vi "Main.vi"() -> ()   [LabVIEW 2017]
doc: "This Continuous Measurement sample project is based on the Queued Message Handler template.\n\nThe Event Handling Loop generates messages based on user interface actions.\n\nThe Message Handling Loop processes messages generated by the Event Handling Loop, or by other messages. There are also Acquisition and Logging message handling loop subVIs, and a chart updating loop."
uses:
  Acquisition/Hardware Configuration.ctl
  Logging/Logging Configuration.ctl
  <vilib>/measure/madcrms.llb/Averaged DC-RMS for 1 Chan.vi
  Feedback.vi
  <vilib>/express/express analysis/Spectral/Block/exnSpectralBlock spectral measurements PSD poly.vi
  <vilib>/express/express analysis/Spectral/Block/exnSpectralBlock spectral measurements PSD DDT.vi
  support/Message Queue/Enqueue Message (Single).vi
  <vilib>/Utility/error.llb/Error Cluster From Error Code.vi
  <vilib>/express/express analysis/Spectral/XNode/ExpressSpectralMeasurementsBlockNode.xnode
  <vilib>/ErrorRing/Error Ring.xnode
  Acquisition/Acquisition.lvlib
  Logging/Logging.lvlib
  Settings/Settings.lvlib
  support/User Event - Stop/User Event - Stop.lvlib
  support/Message Queue/Message Queue.lvlib
  <vilib>/Analysis/NI_AALBase.lvlib
  <vilib>/measure/NI_MAPro.lvlib
panel:
  in  "Average_ON":bool
  in  "Clear":bool
  out "Trap_Power":dbl caption="Trap (V)"
  out "T1Y 2":waveform(dbl)(graph)={"t0"=timestamp(0 s since 1904-01-01), "dt"=1.0, "Y"=[]}
  in  "Reset":bool caption="Offset_Reset"
  out "QPD_x":dbl
  out "QPD_y":dbl
  in  "ON":bool
  in  "B1X_nm2V 2":dbl=1450.0 caption="X"
  in  "B1Y_nm2V 2":dbl=950.0 caption="Y"
  out "Fy":dbl
  out "Fx":dbl caption="F (pN)"
  in  "B1Y_stiffness":dbl=0.1 caption="B1X"
  in  "B1X_stiffness":dbl=0.1 caption="B1X"
  in  "Averaging rate (Hz)":dbl=1000.0 min=1.0 max=1000.0 step=1.0
  in  "Stiffness":bool
  out "B1X PSD":dynamicdata(graph)=[{"t0"=timestamp(0 s since 1904-01-01), "dt"=inf, "Y"=[], "attributes"=variant("NI_ChannelName"=variant(string "Collected (PSD)"), "NI_OriginalChannelName"=variant(string "Collected"))}]
  out "Logging file":path
  out "Stiffness_B1X":dbl
  out "Stiffness_B1Y":dbl
  out "B1S":waveform(dbl)(graph)={"t0"=timestamp(0 s since 1904-01-01), "dt"=1.0, "Y"=[]}
  out "B1X":waveform(dbl)(graph)
  out "B1Y":waveform(dbl)(graph)
  in  "BXY":bool
  out "B1XY":cluster{dbl[], dbl[]}(graph)
  out "T1Y":waveform(dbl)(graph)
  out "T1X":waveform(dbl)(graph)
  out "PZTZ":waveform(dbl)(graph)
  out "PZTY":waveform(dbl)(graph)
  out "PZTX":waveform(dbl)(graph)
  in  "PSD":bool
  in  "B1X_nm2V":dbl=100.0 caption="X"
  in  "B1Y_nm2V":dbl=60.0 caption="Y"
  out "Description":string
  out "User":string
  out "B1Y PSD":dynamicdata(graph)=[{"t0"=timestamp(0 s since 1904-01-01), "dt"=inf, "Y"=[], "attributes"=variant("NI_ChannelName"=variant(string "Collected (PSD)"), "NI_OriginalChannelName"=variant(string "Collected"))}]
  out "Input min (V)":dbl
  out "Input (V)":dbl
  out "Rate (Hz)":dbl
  in  "Stop_Log":bool
  in  "Log":bool
  in  "Exit":bool
  out "?":string
  in  "Settings":bool
  in  "Stop_Acquire":bool
  in  "Acquire":bool
  # "QPD (nm/V)"
  # "k (pN/nm)"
  # "MTA (nm/V)"
  # "Offset (nm)"
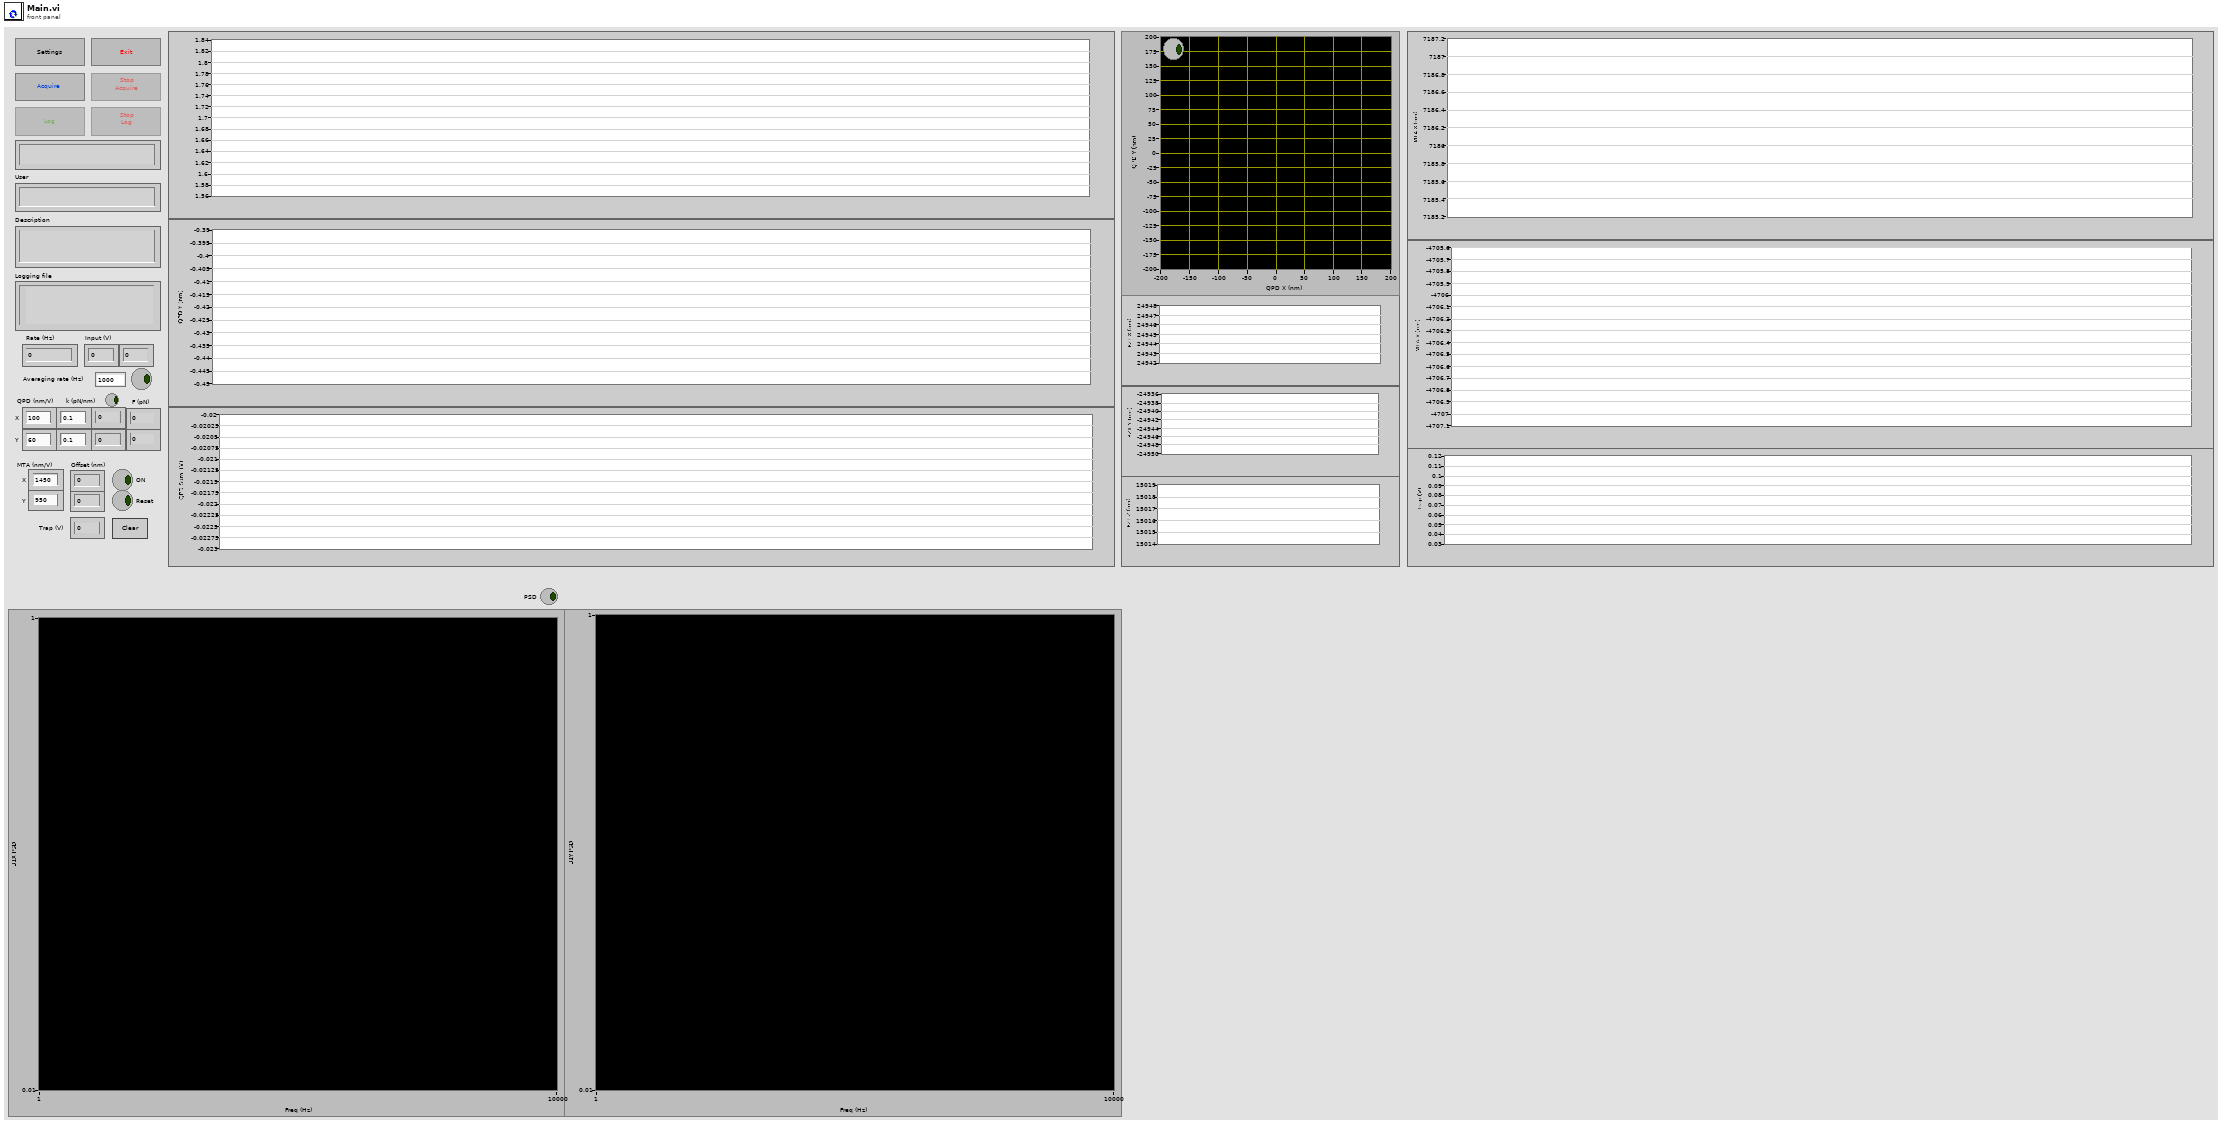
[diagram p1: front panel]
types:
  T1 = cluster{"Acquire Ref":refnum<vi>, "Log Ref":refnum<vi>, "Stop_Acquire Ref":refnum<vi>, "Settings Ref":refnum<vi>, "Status Ref":refnum<vi>, "Exit Ref":refnum<vi>, "Stop_Log Ref":refnum<vi>}
  T2 = typedef "Acquisition.lvlib/Hardware Configuration.ctl" = cluster{"DAQmx Input":tag, "Max Input":dbl, "Min Input":dbl, "Sample Rate":dbl, "DAQmx Task":refnum<k21>}
  T3 = typedef "Logging.lvlib/Logging Configuration.ctl" = cluster{"Log File Base Path":path, "TDMS File Reference":refnum<k34>, "Channel names":string[], "Author":string, "Description":string}
  T4 = cluster{"Hardware Configuration":T2, "Logging Configuration":T3}
  T5 = typedef "Message Queue.lvlib/All Message Queues.ctl" = cluster{"UI":refnum<queue>, "Acquisition":refnum<queue>, "Logging":refnum<queue>}
  T6 = cluster{"Hardware Configuration":T2, "Logging Configuration":cluster{"Log File Base Path":path, "TDMS File Reference":refnum<k34>, "Channel names":string[], "Author":string, "Description":string}}
  T7 = cluster{"averaging mode":u16, "weighting mode":u16, "number of averages":u32}
  T8 = cluster{"dB On (F)":bool, "unwrap phase (F)":bool, "convert to degree (F)":bool}
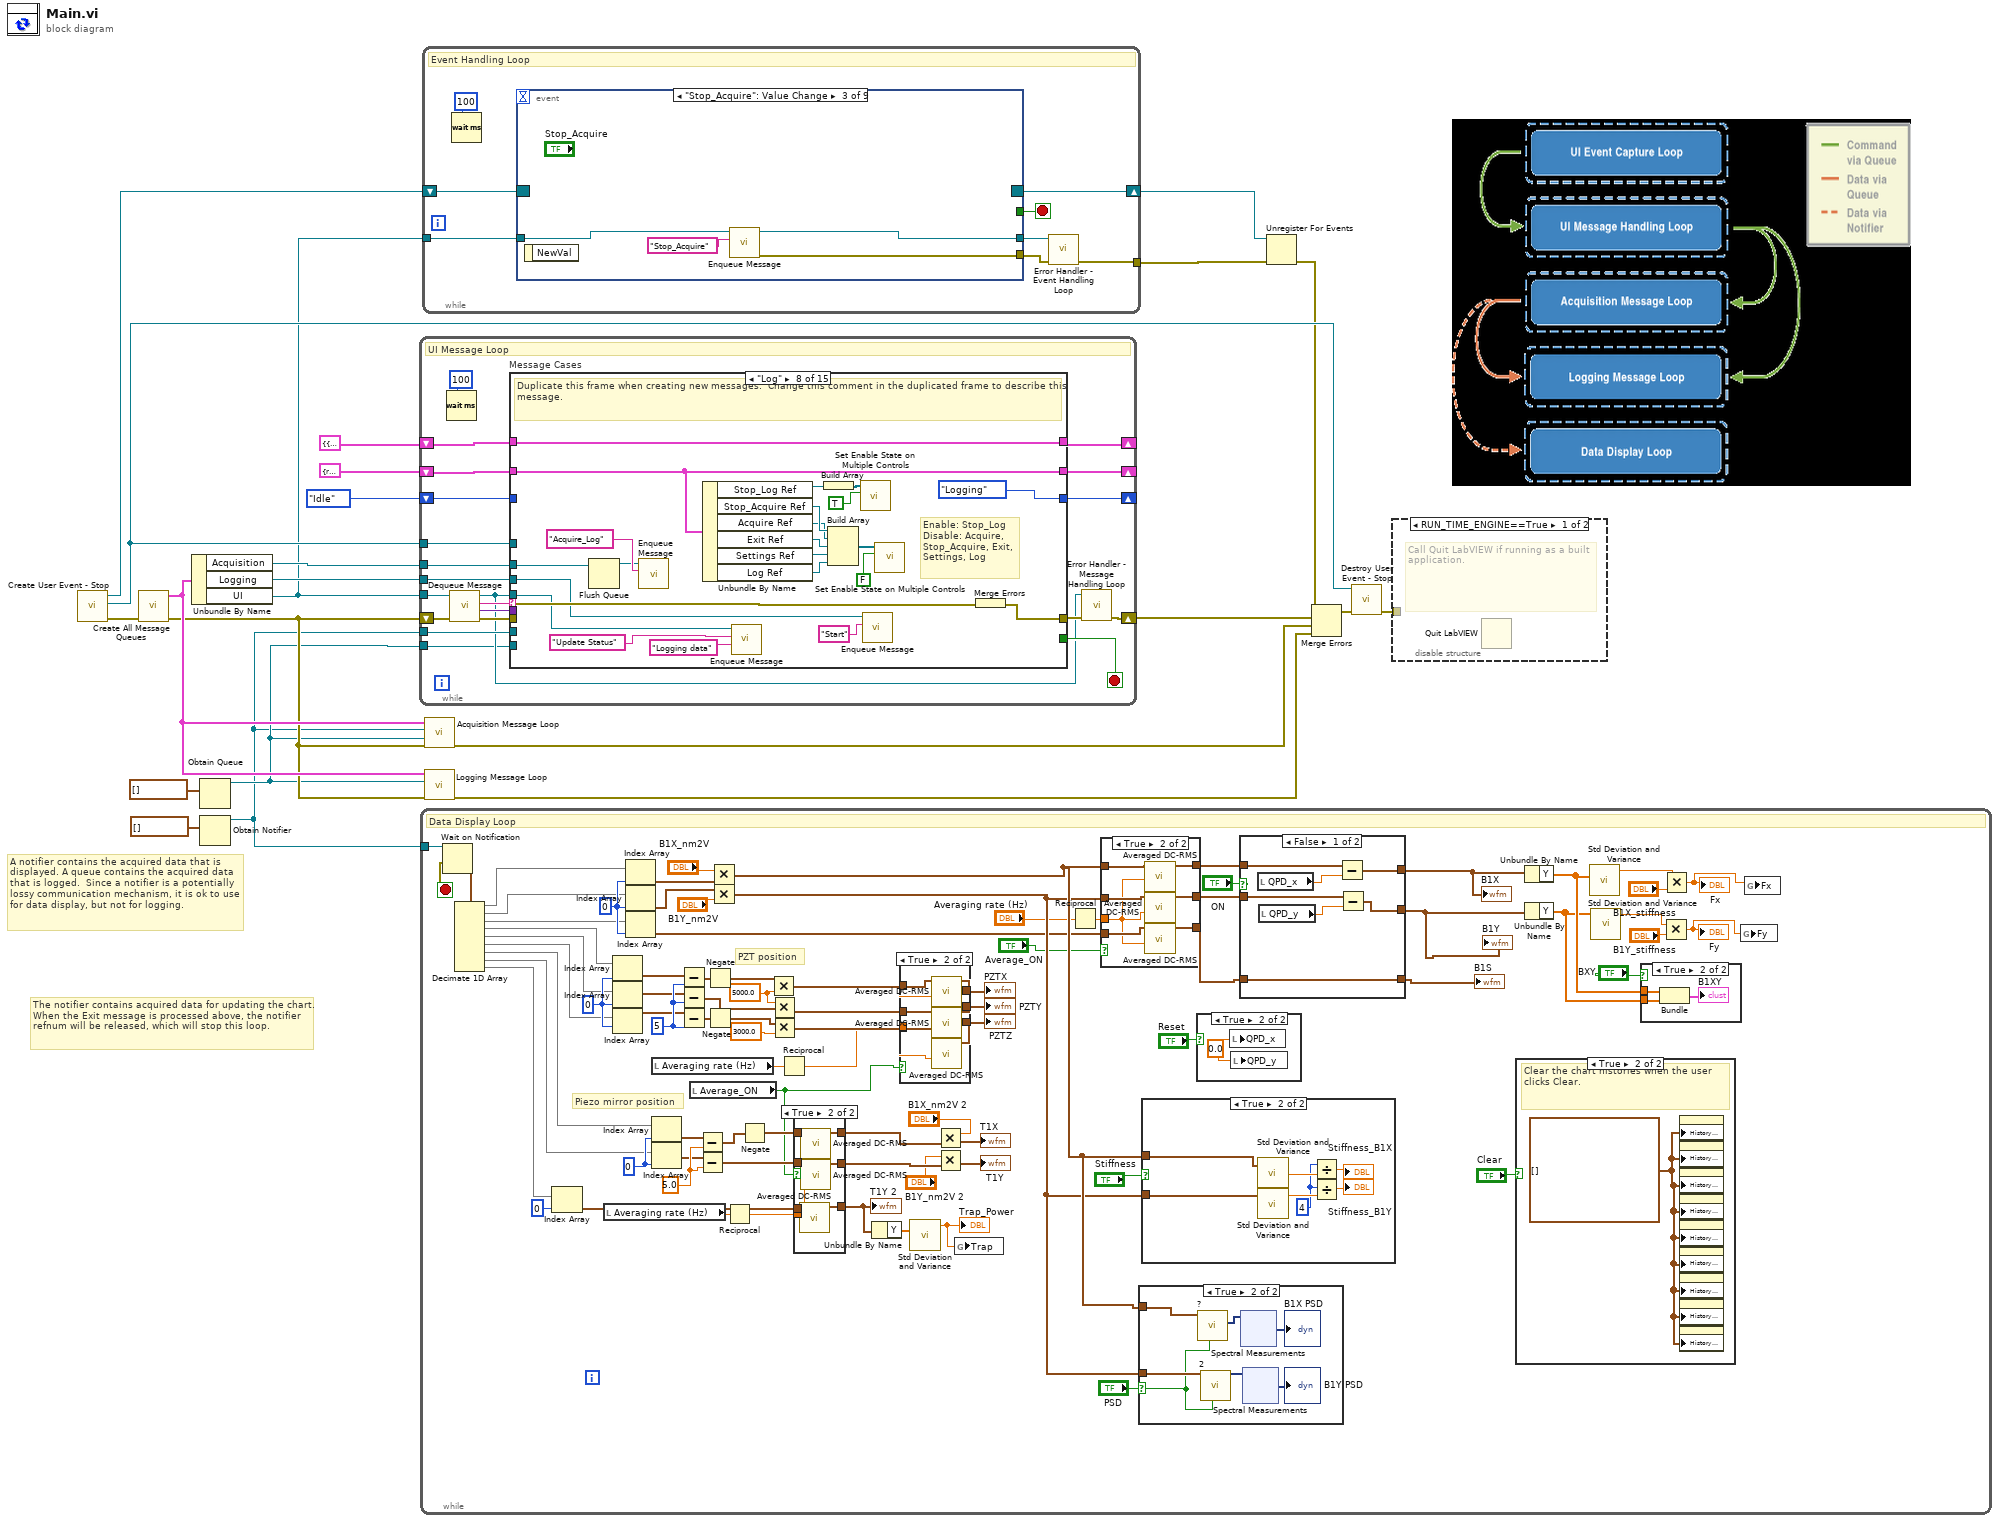
[diagram p0: block diagram]
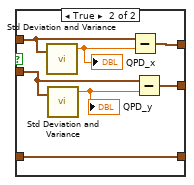
[diagram p8: hidden frame]
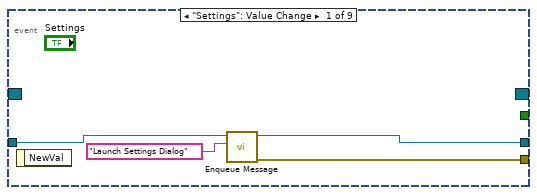
[diagram p12: hidden frame]
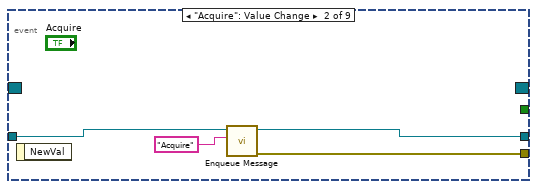
[diagram p13: hidden frame]
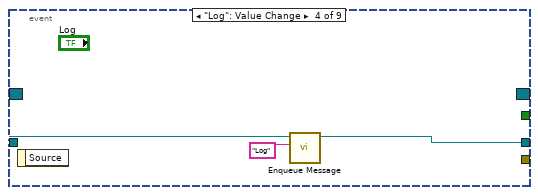
[diagram p14: hidden frame]
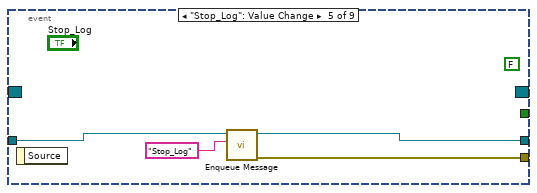
[diagram p15: hidden frame]
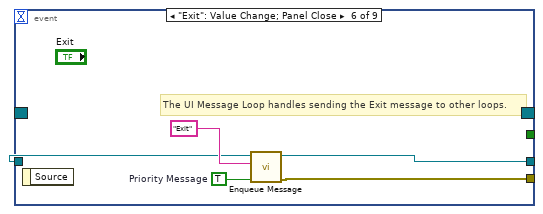
[diagram p16: hidden frame]
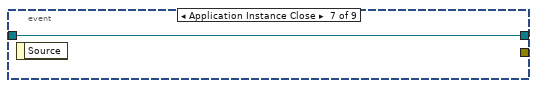
[diagram p17: hidden frame]
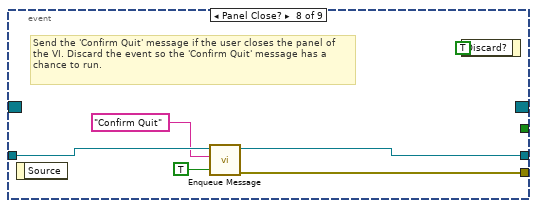
[diagram p18: hidden frame]
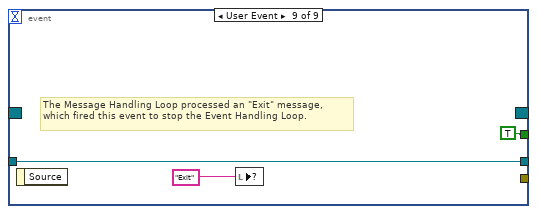
[diagram p19: hidden frame]
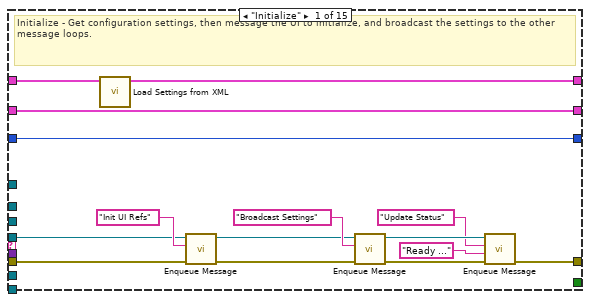
[diagram p20: hidden frame]
diagram:
  # "A notifier contains the acquired data that is displayed. A queue contains the acquired data that is logged.  Since a notifier is a potentially lossy communication mechanism, it is ok to use for data display, but not for logging."
  # "The notifier contains acquired data for updating the chart. When the Exit message is processed above, the notifier refnum will be released, which will stop this loop."
  n1 = call "Create User Event - Stop.vi"() -> ("error out"=w17:errorcluster, "User Event - Stop"=w19:refnum<user-event>, "Stop Event Registration Refnum"=w20:refnum<event-registration>)  [unwired: 9 in]
  n2 = call "Create All Message Queues.vi"("error in (no error)"=w17) -> ("error out"=w4:errorcluster, "Message Queues out"=w16:T5)  [unwired: 9 in]
  n3 = Unbundle By Name(w16) -> ("Acquisition"=w11:refnum<queue>, "Logging"=w10:refnum<queue>, "UI"=w3:refnum<queue>)
  n4 = Obtain Queue(element data type=waveform(sgl)[] []) -> (queue out=w2:refnum<queue>)  [unwired: 4 in, 2 out]
  n5 = Obtain Notifier(notification data type=waveform(sgl)[] []) -> (notifier out=w1:refnum<notifier>)  [unwired: 3 in, 2 out]
  n6 = while {
    tunnel: w3 -> [w38]
    tunnel: w19 -> [w43]
    shift-right: [w31] -> w23
    shift-left: w4 -> [w42]
    shift-right: [w29] -> _
    shift-left: T4 {"Hardware Configuration"={"DAQmx Input"="", "Max Input"=0.0, "Min Input"=0.0, "Sample Rate"=0.0, "DAQmx Task"=""}, "Logging Configuration"={"Log File Base Path"=path "", "TDMS File Reference"=refnum, "Channel names"=[], "Author"="", "Description"=""}} ("Settings") -> [w25]
    shift-right: [w36] -> _
    shift-left: T1 {"Acquire Ref"=refnum, "Log Ref"=refnum, "Stop_Acquire Ref"=refnum, "Settings Ref"=refnum, "Status Ref"=refnum, "Exit Ref"=refnum, "Stop_Log Ref"=refnum} ("Measurement UI Controls") -> [w37]
    tunnel: w11 -> [w35]
    tunnel: w10 -> [w34]
    tunnel: w1 -> [w33]
    shift-right: [w28] -> _
    shift-left: enum16{"Idle", "Acquiring", "Logging"}."Idle" ("UI State") -> [w27]
    tunnel: w2 -> [w26]
    stop <- w44 stop-if-true
    # "UI Message Loop"
    n7 = Wait (ms)(milliseconds to wait=u32 100) -> ()  [unwired: 1 out]
    n8 = call "Dequeue Message.vi"("error in (no error)"=w42, "Message Queue"=w38) -> ("error out"=w41:errorcluster, "Message Data"=w39:variant, "Message"=w40:string, "dup Message Queue"=w30:refnum<queue>)  [unwired: 6 in]
    n9 = case "Message Cases" shown="\"Log\"" w40 {
      selector: w40 -> [_ _ _ _ _ _ _ _ _ _ _ _ _ _ w295]
      tunnel: w30 -> [w51 _ w82 _ w107 w135 w140 w180 w186 w215 w233 w271 _ _ _]
      tunnel: w41 -> [w50 w76 w80 w99 w109 w117 w142 w182 w205 w222 w230 w275 w281 w292 _]
      tunnel: [w57 w76 w91 w100 w105 w136 w159 w181 w204 w223 w229 w266 w280 w291 w296] -> w32
      tunnel: [_ _ _ _ _ _ _ _ _ TRUE _ _ _ _ _] -> w44
      tunnel: w39 -> [_ _ _ w98 _ _ _ _ _ _ _ w274 _ _ _]
      tunnel: w43 -> [_ _ _ _ _ _ _ _ _ w221 _ _ _ _ _]
      tunnel: w25 -> [w47 w61 w78 w93 w103 w116 w144 w164 w190 w208 w227 w265 w278 w286 w294]
      tunnel: w37 -> [w53 w75 w85 w95 w104 w132 w158 w177 w203 w218 w234 w276 w279 w290 w297]
      tunnel: [w53 w74 w85 w95 w104 w132 w158 w177 w203 w218 w234 w276 w279 w290 w297] -> w36
      tunnel: w35 -> [_ _ w84 _ _ w123 w154 w162 w188 w217 w232 _ _ _ _]
      tunnel: w34 -> [_ _ w83 _ _ _ _ w174 w200 w216 w231 _ _ _ _]
      tunnel: w33 -> [_ _ _ _ _ _ _ _ _ w214 _ _ _ _ _]
      tunnel: [w46 w61 w78 w93 w102 w116 w144 w164 w190 w208 w227 w265 w278 w286 w294] -> w29
      tunnel: [w45 w60 w77 w92 w101 enum16{"Idle", "Acquiring", "Logging"}."Acquiring" ("UI State") enum16{"Idle", "Acquiring", "Logging"}."Idle" ("UI State") enum16{"Idle", "Acquiring", "Logging"}."Logging" ("UI State") enum16{"Idle", "Acquiring", "Logging"}."Acquiring" ("UI State") enum16{"Idle", "Acquiring", "Logging"}."Idle" ("UI State") w226 w264 w277 w283 w293] -> w28
      tunnel: w27 -> [w45 w60 w77 w92 w101 _ _ _ _ _ w225 w264 w277 w283 w293]
      tunnel: w26 -> [_ _ _ _ _ _ _ _ _ w206 _ _ _ _ _]
      frame "Initialize" {
        # "Initialize - Get configuration settings, then message the UI to initialize, and broadcast the settings to the other message loops."
        n10 = call "Load Settings from XML.vi"("Settings in"=w47) -> ("Settings out"=w46:T4)  [unwired: 9 in, 1 out]
        n11 = call-poly "Enqueue Message.vi"("error in (no error)"=w50, "Message"="Init UI Refs", "Message Queue"=w51) -> ("error out"=w48:errorcluster, "dup Message Queue"=w49:refnum<queue>)  [unwired: 7 in]
        n12 = call-poly "Enqueue Message.vi"("error in (no error)"=w48, "Message"="Broadcast Settings", "Message Queue"=w49) -> ("error out"=w59:errorcluster, "dup Message Queue"=w58:refnum<queue>)  [unwired: 7 in]
        n13 = call-poly "Enqueue Message.vi"("error in (no error)"=w59, "Message Data"="Ready ..." ("Ready..."), "Message"="Update Status", "Message Queue"=w58) -> ("error out"=w57:errorcluster)  [unwired: 6 in, 1 out]
      }
      frame "Init UI Refs" {
        # "Stop_Log"
        # "Enable: Acquire, Exit, Settings\nDisable: Stop_Acquire, Log, Stop_Log"
        # "Init UI Refs - Store control references for UI controls.  Also enable/disable controls appropriately."
        n14 = property class="VI"("Front Panel.Closeable"=TRUE ("Front Panel Window:Closeable")) -> ()  [unwired: 2 in, 2 out]
        n15 = control-ref of="Acquire"() -> (w70:refnum<vi>)
        n16 = control-ref of="Log"() -> (w66:refnum<vi>)
        n17 = control-ref of="Stop_Acquire"() -> (w65:refnum<vi>)
        n18 = control-ref of="Settings"() -> (w67:refnum<vi>)
        n19 = control-ref of="Exit"() -> (w63:refnum<vi>)
        n20 = control-ref of="?"() -> (w62:refnum<vi>)
        n21 = control-ref of="?"() -> (w71:refnum<vi>)
        n22 = Build Array(w63, w67, w70) -> (w69:refnum<vi>[])
        n23 = Bundle By Name(cluster=w75, "Acquire Ref"=w70, "Log Ref"=w66, "Stop_Acquire Ref"=w65, "Settings Ref"=w67, "Status Ref"=w71, "Exit Ref"=w63, "Stop_Log Ref"=w62) -> (w74:T1)
        n24 = Build Array(w65, w66, w62) -> (w64:refnum<vi>[])
        n25 = call "Set Enable State on Multiple Controls.vi"("Enable?"=TRUE, "Controls"=w69) -> ()  [unwired: 10 in]
        n26 = call "Set Enable State on Multiple Controls.vi"("Enable?"=FALSE, "Controls"=w64) -> ()  [unwired: 10 in]
      }
      frame "Broadcast settings" {
        w86 = "Update Settings" ("Message")
        # "Send the 'Update Settings' message to the Logging and Acquisition message loops."
        n27 = Unbundle By Name(w78) -> ("Hardware Configuration"=w89:T2, "Logging Configuration"=w88:T3)
        n28 = call-poly "Enqueue Message.vi"("error in (no error)"=w80, "Message"="Display Setting", "Message Queue"=w82) -> ("error out"=w79:errorcluster)  [unwired: 7 in, 1 out]
        n29 = call-poly "Enqueue Message.vi"("Message Data"=w89, "Message"=w86, "Message Queue"=w84) -> ("error out"=w90:errorcluster)  [unwired: 7 in, 1 out]
        n30 = call-poly "Enqueue Message.vi"("error in (no error)"=w90, "Message Data"=w88, "Message"=w86, "Message Queue"=w83) -> ("error out"=w87:errorcluster)  [unwired: 6 in, 1 out]
        n31 = Merge Errors(w87, w80, w79) -> (w91:errorcluster)
      }
      frame "Update Status" {
        # "Update Display - Convert the message data to a string to display in the Status indicator."
        n32 = Variant To Data(error in=w99, type="", Variant=w98) -> (data=→"?":string, error out=w96:errorcluster)
        n33 = Merge Errors(w96) -> (w100:errorcluster)
      }
      frame "Launch Settings Dialog" {
        # "Launch the Settings Dialog when the user clicks the 'Settings' button."
        n34 = call "Settings Dialog.vi"("error in (no error)"=w109, "Settings in"=w103) -> ("error out"=w106:errorcluster, "Cancelled?"=w108:bool, "Settings out"=w102:T6)  [unwired: 6 in, 1 out]
        n35 = case shown="False" w108 {
          tunnel: w107 -> [w113 _]
          tunnel: w106 -> [w112 w114]
          tunnel: [w111 w114] -> w105
          frame False {
            n36 = call-poly "Enqueue Message.vi"("error in (no error)"=w112, "Message"="Broadcast Settings", "Message Queue"=w113) -> ("error out"=w111:errorcluster)  [unwired: 7 in, 1 out]
          }
          frame True {
          }
        }
      }
      frame "Acquire" {
        # "Message Acquisition loops to start"
        # "Enable: Stop_Acquire, Log\nDisable: Acquire, Stop_Log, Exit, Settings"
        # "Start - Enable/Disable buttons appropriately for an acquisition that has started, and update status display."
        n37 = Unbundle By Name(w132) -> ("Log Ref"=w120:refnum<vi>, "Stop_Acquire Ref"=w121:refnum<vi>, "Acquire Ref"=w127:refnum<vi>, "Exit Ref"=w126:refnum<vi>, "Settings Ref"=w125:refnum<vi>, "Stop_Log Ref"=w118:refnum<vi>)
        n38 = call-poly "Enqueue Message.vi"("error in (no error)"=w117, "Message Data"="Acquiring data" ("Waiting for trigger"), "Message"="Update Status", "Message Queue"=w135) -> ("error out"=w119:errorcluster)  [unwired: 6 in, 1 out]
        n39 = Build Array(w127, w126, w125, w118) -> (w130:refnum<vi>[])
        n40 = Build Array(w120, w121) -> (w129:refnum<vi>[])
        n41 = call "Set Enable State on Multiple Controls.vi"("Enable?"=TRUE, "Controls"=w129) -> ()  [unwired: 10 in]
        n42 = call "Set Enable State on Multiple Controls.vi"("Enable?"=FALSE, "Controls"=w130) -> ()  [unwired: 10 in]
        n43 = call-poly "Enqueue Message.vi"("error in (no error)"=w119, "Message"="Start", "Message Queue"=w123) -> ("error out"=w124:errorcluster)  [unwired: 7 in, 1 out]
        n44 = Merge Errors(w124) -> (w136:errorcluster)
      }
      frame "Stop_Acquire" {
        # "Message Acquisition loop to stop"
        # "Enable: Acquire, Exit, Settings\nDisable: Stop_Acquire, Log, Stop_Log"
        # "Stop - Enable/Disable buttons appropriately for an acquisition that has stopped, and update status display."
        n45 = Unbundle By Name(w158) -> ("Log Ref"=w152:refnum<vi>, "Stop_Acquire Ref"=w151:refnum<vi>, "Acquire Ref"=w150:refnum<vi>, "Exit Ref"=w149:refnum<vi>, "Settings Ref"=w148:refnum<vi>, "Stop_Log Ref"=w147:refnum<vi>)
        n46 = call-poly "Enqueue Message.vi"("error in (no error)"=w142, "Message Data"="Ready..." ("Message"), "Message"="Update Status", "Message Queue"=w140) -> ("error out"=w141:errorcluster)  [unwired: 6 in, 1 out]
        n47 = Build Array(w152, w151, w147) -> (w145:refnum<vi>[])
        n48 = Build Array(w150, w149, w148) -> (w146:refnum<vi>[])
        n49 = call "Set Enable State on Multiple Controls.vi"("Enable?"=TRUE, "Controls"=w146) -> ()  [unwired: 10 in]
        n50 = call "Set Enable State on Multiple Controls.vi"("Enable?"=FALSE, "Controls"=w145) -> ()  [unwired: 10 in]
        n51 = call-poly "Enqueue Message.vi"("Priority Message? (F)"=TRUE, "error in (no error)"=w141, "Message"="Stop", "Message Queue"=w154) -> ("error out"=w155:errorcluster)  [unwired: 6 in, 1 out]
        n52 = Merge Errors(w155) -> (w159:errorcluster)
      }
      frame "Log" {
        # "Enable: Stop_Log\nDisable: Acquire, Stop_Acquire, Exit, Settings, Log"
        # "Duplicate this frame when creating new messages.  Change this comment in the duplicated frame to describe this message."
        n53 = Flush Queue(queue=w162) -> (queue out=w161:refnum<queue>)  [unwired: 1 in, 2 out]
        n54 = call-poly "Enqueue Message.vi"("Message"="Acquire_Log", "Message Queue"=w161) -> ()  [unwired: 8 in, 2 out]
        n55 = Unbundle By Name(w177) -> ("Stop_Log Ref"=w172:refnum<vi>, "Stop_Acquire Ref"=w170:refnum<vi>, "Acquire Ref"=w169:refnum<vi>, "Exit Ref"=w168:refnum<vi>, "Settings Ref"=w167:refnum<vi>, "Log Ref"=w166:refnum<vi>)
        n56 = call-poly "Enqueue Message.vi"("Message Data"="Logging data" ("Ready..."), "Message"="Update Status", "Message Queue"=w180) -> ()  [unwired: 7 in, 2 out]
        n57 = Build Array(w172) -> (w171:refnum<vi>[])
        n58 = Build Array(w170, w169, w168, w167, w166) -> (w165:refnum<vi>[])
        n59 = call "Set Enable State on Multiple Controls.vi"("Enable?"=TRUE, "Controls"=w171) -> ()  [unwired: 10 in]
        n60 = call-poly "Enqueue Message.vi"("Message"="Start", "Message Queue"=w174) -> ()  [unwired: 8 in, 2 out]
        n61 = call "Set Enable State on Multiple Controls.vi"("Enable?"=FALSE, "Controls"=w165) -> ()  [unwired: 10 in]
        n62 = Merge Errors(w182) -> (w181:errorcluster)
      }
      frame "Stop_Log" {
        # "Message Logging loop to stop"
        # "Enable: Log, Stop_Acquire\nDisable: Acquire, Exit, Settings, Stop_Log"
        # "Duplicate this frame when creating new messages.  Change this comment in the duplicated frame to describe this message."
        n63 = Flush Queue(queue=w188) -> (queue out=w187:refnum<queue>)  [unwired: 1 in, 2 out]
        n64 = call-poly "Enqueue Message.vi"("Message"="Acquire", "Message Queue"=w187) -> ()  [unwired: 8 in, 2 out]
        n65 = call-poly "Enqueue Message.vi"("Message"="Stop", "Message Queue"=w200) -> ()  [unwired: 8 in, 2 out]
        n66 = call-poly "Enqueue Message.vi"("Message Data"="Acquiring data" ("Ready..."), "Message"="Update Status", "Message Queue"=w186) -> ()  [unwired: 7 in, 2 out]
        n67 = Unbundle By Name(w203) -> ("Stop_Acquire Ref"=w198:refnum<vi>, "Log Ref"=w192:refnum<vi>, "Acquire Ref"=w196:refnum<vi>, "Exit Ref"=w195:refnum<vi>, "Settings Ref"=w194:refnum<vi>, "Stop_Log Ref"=w191:refnum<vi>)
        n68 = Build Array(w198, w192) -> (w197:refnum<vi>[])
        n69 = Build Array(w191, w196, w195, w194) -> (w193:refnum<vi>[])
        n70 = call "Set Enable State on Multiple Controls.vi"("Enable?"=TRUE, "Controls"=w197) -> ()  [unwired: 10 in]
        n71 = call "Set Enable State on Multiple Controls.vi"("Enable?"=FALSE, "Controls"=w193) -> ()  [unwired: 10 in]
        n72 = Merge Errors(w205) -> (w204:errorcluster)
      }
      frame "Exit" {
        w219 = "Exit" ("Message")
        # "Stop the VI"
        # "Exit - Fire the User Event to stop the Event Handling Loop.  Also send Exit messages to the Acquisition and Logging loops."
        n73 = Release Queue(queue=w215, error in (no error)=w222) -> (error out=w213:errorcluster)  [unwired: 1 in, 2 out]
        n74 = call "Fire User Event - Stop.vi"("User Event - Stop"=w221) -> ("error out"=w220:errorcluster)  [unwired: 10 in]
        n75 = Release Notifier(notifier=w214, error in (no error)=w213) -> (error out=w212:errorcluster)  [unwired: 1 in, 2 out]
        n76 = call-poly "Enqueue Message.vi"("Priority Message? (F)"=TRUE, "Message"=w219, "Message Queue"=w217) -> ()  [unwired: 7 in, 2 out]
        n77 = Release Queue(queue=w206, error in (no error)=w212) -> (error out=w211:errorcluster)  [unwired: 1 in, 2 out]
        n78 = call-poly "Enqueue Message.vi"("Priority Message? (F)"=TRUE, "Message"=w219, "Message Queue"=w216) -> ()  [unwired: 7 in, 2 out]
        n79 = Merge Errors(w220, w211) -> (w223:errorcluster)
      }
      frame "Confirm Quit" {
        # "Confirm Quit - Message that can confirm whether or not the user wants to exit the application."
        n80 = while {
          tunnel: w233 -> [w243]
          tunnel: w232 -> [w242]
          tunnel: w231 -> [w241]
          shift-right: [w237] -> w228
          shift-left: w230 -> [w240]
          shift-right: [w239] -> w226
          shift-left: w225 -> [w238]
          stop <- w236 stop-if-true
          n81 = case shown="\"Logging\"" w238 {
            selector: w238 -> [w245 _ _]
            tunnel: [w247 w250 w258] -> w237
            tunnel: [w245 enum16{"Idle", "Acquiring", "Logging"}."Idle" ("UI State") enum16{"Idle", "Acquiring", "Logging"}."Acquiring" ("UI State")] -> w239
            tunnel: w243 -> [w246 _ _]
            tunnel: w242 -> [_ w254 _]
            tunnel: w240 -> [_ w251 w257]
            tunnel: w241 -> [_ _ w263]
            tunnel: [TRUE ("Priority Message? (F)") FALSE ("Priority Message? (F)") FALSE ("Priority Message? (F)")] -> w236
            frame "Idle", Default {
              n82 = call-poly "Enqueue Message.vi"("Priority Message? (F)"=TRUE, "Message"="Exit", "Message Queue"=w246) -> ("error out"=w247:errorcluster)  [unwired: 7 in, 1 out]
            }
            frame "Acquiring" {
              n83 = call-poly "Enqueue Message.vi"("Priority Message? (F)"=TRUE, "error in (no error)"=w251, "Message"="Stop", "Message Queue"=w254) -> ("error out"=w250:errorcluster)  [unwired: 6 in, 1 out]
            }
            frame "Logging" {
              n84 = call-poly "Enqueue Message.vi"("Priority Message? (F)"=TRUE, "error in (no error)"=w257, "Message"="Stop", "Message Queue"=w263) -> ("error out"=w258:errorcluster)  [unwired: 6 in, 1 out]
            }
          }
          n85 = Wait (ms)(milliseconds to wait=u32 100) -> ()  [unwired: 1 out]
        }
        n86 = Merge Errors(w228, w230) -> (w229:errorcluster)
      }
      frame "Error" {
        # "Error - Check the error message data and respond accordingly. This message is sent by the \"Error Handler\" VIs at the end of each loop in this application."
        n87 = Variant To Data(error in=w275, type=errorcluster {"status"=FALSE, "code"=0, "source"=""} ("error out"), Variant=w274) -> (data=w272:errorcluster, error out=w268:errorcluster)
        n88 = call <vilib>:"Simple Error Handler.vi"("error in (no error)"=w272) -> ()  [unwired: 4 in, 5 out]
        n89 = call-poly "Enqueue Message.vi"("Priority Message? (F)"=TRUE, "Message"="Exit", "Message Queue"=w271) -> ("error out"=w267:errorcluster)  [unwired: 7 in, 1 out]
        n90 = Merge Errors(w267, w268) -> (w266:errorcluster)
      }
      frame "---Copy This Frame---" {
        # "Duplicate this frame when creating new messages.  Change this comment in the duplicated frame to describe this message."
        n91 = Merge Errors(w281) -> (w280:errorcluster)
      }
      frame "Display Setting" {
        # "Duplicate this frame when creating new messages.  Change this comment in the duplicated frame to describe this message."
        n92 = Unbundle By Name(w286) -> ("Hardware Configuration.Sample Rate"=→"Rate (Hz)":dbl, "Hardware Configuration.Max Input"=→"Input (V)":dbl, "Hardware Configuration.Min Input"=→"Input min (V)":dbl, "Logging Configuration.Author"=→"User":string, "Logging Configuration.Description"=→"Description":string, "Logging Configuration.Log File Base Path"=→"Logging file":path)
        n93 = Merge Errors(w292) -> (w291:errorcluster)
      }
      frame Default {
        # "'Default' case only runs if there is a message that isn't defined in any of the other cases.  Output a programming error."
        n94 = xnode "Error Ring"("parameter 0"=w295) -> ("error out"=w296:errorcluster)
      }
    }
    n95 = call "Error Handler - Message Handling Loop.vi"("error in (no error)"=w32, "Message Queue"=w30) -> ("dup error in"=w31:errorcluster)  [unwired: 8 in, 1 out]
  }
  n96 = while "Data Display Loop" {
    tunnel: w1 -> [w388]
    stop <- w384 stop-if-true
    w371 = 5
    w377 = 0 ("index")
    w378 = 0 ("index")
    w379 = 5.0 ("x")
    w380 = 0 ("index")
    w372 = 5000.0 ("y")
    # "Piezo mirror position"
    # "PZT position"
    # "Data Display Loop"
    n97 = Wait on Notification(notifier=w388) -> (notification=w387:waveform(sgl)[], error out=w384:errorcluster)  [unwired: 3 in, 2 out]
    n98 = Decimate 1D Array(w387) -> (w376:waveform(sgl)[], w375:waveform(sgl)[], w374:waveform(sgl)[], w360:waveform(sgl)[], w359:waveform(sgl)[], w358:waveform(sgl)[], w357:waveform(sgl)[], w356:waveform(sgl)[], w313:waveform(sgl)[])
    n99 = Index Array(array=w313, index=0) -> (element=w311:waveform(sgl))
    n100 = local read "Averaging rate (Hz)"() -> (w338:dbl)
    n101 = Index Array(array=w360, index=w378) -> (element=w365:waveform(sgl))
    n102 = Index Array(array=w359, index=w378) -> (element=w364:waveform(sgl))
    n103 = Index Array(array=w358, index=w378) -> (element=w363:waveform(sgl))
    n104 = Index Array(array=w376, index=w377) -> (element=w367:waveform(sgl))
    n105 = Index Array(array=w375, index=w377) -> (element=w366:waveform(sgl))
    n106 = Index Array(array=w374, index=w377) -> (element=w351:waveform(sgl))
    n107 = local read "Averaging rate (Hz)"() -> (w346:dbl)
    n108 = Index Array(array=w357, index=w380) -> (element=w362:waveform(sgl))
    n109 = Index Array(array=w356, index=w380) -> (element=w361:waveform(sgl))
    n110 = Subtract(x=w365, y=w371) -> (x-y=w383:waveform(sgl))
    n111 = Subtract(x=w364, y=w371) -> (x-y=w369:waveform(sgl))
    n112 = Subtract(x=w363, y=w371) -> (x-y=w382:waveform(sgl))
    n113 = local read "Average_ON"() -> (w305:bool)
    n114 = Subtract(x=w362, y=w379) -> (x-y=w342:waveform(dbl))
    n115 = Subtract(x=w361, y=w379) -> (x-y=w341:waveform(dbl))
    n116 = Negate(x=w383) -> (-x=w370:waveform(sgl))
    n117 = Negate(x=w382) -> (-x=w368:waveform(sgl))
    n118 = Multiply(x="B1X_nm2V", y=w367) -> (x*y=w353:waveform(dbl))
    n119 = Multiply(x=w366, y="B1Y_nm2V") -> (x*y=w352:waveform(dbl))
    n120 = Reciprocal(x=w338) -> (1/x=w317:dbl)
    n121 = Negate(x=w342) -> (-x=w327:waveform(dbl))
    n122 = Multiply(x=w370, y=w372) -> (x*y=w349:waveform(dbl))
    n123 = Multiply(x=w372, y=w369) -> (x*y=w348:waveform(dbl))
    n124 = Multiply(x=w368, y=3000.0) -> (x*y=w347:waveform(dbl))
    n125 = Reciprocal(x=w346) -> (1/x=w336:dbl)
    n126 = case shown="True" w305 {
      tunnel: w341 -> [w390 w398]
      tunnel: [w391 w397] -> w340
      tunnel: [w390 w396] -> w339
      tunnel: w327 -> [w391 w395]
      tunnel: w317 -> [_ w394]
      tunnel: [w389 w393] -> w314
      tunnel: w311 -> [w389 w392]
      frame False {
      }
      frame True {
        n127 = call-poly <vilib>:"Averaged DC-RMS.vi"("averaging time"=w394, "signal in"=w392) -> ("DC value waveform"=w393:waveform(dbl))  [unwired: 5 in, 4 out]
        n128 = call-poly <vilib>:"Averaged DC-RMS.vi"("averaging time"=w394, "signal in"=w395) -> ("DC value waveform"=w397:waveform(dbl))  [unwired: 5 in, 4 out]
        n129 = call-poly <vilib>:"Averaged DC-RMS.vi"("averaging time"=w394, "signal in"=w398) -> ("DC value waveform"=w396:waveform(dbl))  [unwired: 5 in, 4 out]
      }
    }
    "T1Y 2" <- w314
    n130 = Unbundle By Name(w314) -> ("Y"=w316:dbl[])
    n131 = case shown="True" w305 {
      tunnel: w349 -> [w401 w408]
      tunnel: w348 -> [w400 w407]
      tunnel: w347 -> [w399 w406]
      tunnel: [w401 w405] -> w345
      tunnel: [w400 w404] -> w344
      tunnel: [w399 w403] -> w343
      tunnel: w336 -> [_ w402]
      frame False {
      }
      frame True {
        n132 = call-poly <vilib>:"Averaged DC-RMS.vi"("averaging time"=w402, "signal in"=w408) -> ("DC value waveform"=w405:waveform(dbl))  [unwired: 5 in, 4 out]
        n133 = call-poly <vilib>:"Averaged DC-RMS.vi"("averaging time"=w402, "signal in"=w407) -> ("DC value waveform"=w404:waveform(dbl))  [unwired: 5 in, 4 out]
        n134 = call-poly <vilib>:"Averaged DC-RMS.vi"("averaging time"=w402, "signal in"=w406) -> ("DC value waveform"=w403:waveform(dbl))  [unwired: 5 in, 4 out]
      }
    }
    "PZTX" <- w345
    "PZTY" <- w344
    "PZTZ" <- w343
    n135 = call <vilib>:"Std Deviation and Variance.vi"("X"=w316) -> ("mean"=w315:dbl)  [unwired: 1 in, 2 out]
    "Trap_Power" <- w315
    n136 = Multiply(x="B1X_nm2V 2", y=w340) -> (x*y=→"T1X":waveform(dbl))
    n137 = Multiply(x="B1Y_nm2V 2", y=w339) -> (x*y=→"T1Y":waveform(dbl))
    n138 = global write "Feedback.vi" "Trap"(w315) -> ()
    n139 = Reciprocal(x="Averaging rate (Hz)") -> (1/x=w337:dbl)
    n140 = case shown="True" "Average_ON" {
      tunnel: w353 -> [w411 w418]
      tunnel: w352 -> [w410 w417]
      tunnel: w351 -> [w409 w416]
      tunnel: w337 -> [_ w415]
      tunnel: [w410 w414] -> w324
      tunnel: [w411 w413] -> w323
      tunnel: [w409 w412] -> w308
      frame False {
      }
      frame True {
        n141 = call-poly <vilib>:"Averaged DC-RMS.vi"("averaging time"=w415, "signal in"=w418) -> ("DC value waveform"=w413:waveform(dbl))  [unwired: 5 in, 4 out]
        n142 = call-poly <vilib>:"Averaged DC-RMS.vi"("averaging time"=w415, "signal in"=w417) -> ("DC value waveform"=w414:waveform(dbl))  [unwired: 5 in, 4 out]
        n143 = call-poly <vilib>:"Averaged DC-RMS.vi"("averaging time"=w415, "signal in"=w416) -> ("DC value waveform"=w412:waveform(dbl))  [unwired: 5 in, 4 out]
      }
    }
    n144 = case shown="True" "PSD" {
      selector: "PSD" -> [_ w442]
      tunnel: w353 -> [_ w446]
      tunnel: w352 -> [_ w445]
      frame False {
      }
      frame True {
        n145 = call "?"("Reset"=w442, "Signals"=w446) -> ("Collected Signals"=w444:dynamicdata)  [unwired: 8 in, 1 out]
        n146 = call "2"("Reset"=w442, "Signals"=w445) -> ("Collected Signals"=w443:dynamicdata)  [unwired: 8 in, 1 out]
        n147 = xnode ("Spectral Measurements")("Signals"=w444) -> ("PSD"=→"B1X PSD":dynamicdata)  [unwired: 2 in, 2 out]
        n148 = xnode ("Spectral Measurements")("Signals"=w443) -> ("PSD"=→"B1Y PSD":dynamicdata)  [unwired: 2 in, 2 out]
      }
    }
    n149 = case shown="True" "Stiffness" {
      tunnel: w353 -> [_ w436]
      tunnel: w352 -> [_ w435]
      frame False {
      }
      frame True {
        w437 = 4
        n150 = call <vilib>:"Std Deviation and Variance.vi"("X"=w436) -> ("variance"=w439:dbl)  [unwired: 1 in, 2 out]
        n151 = call <vilib>:"Std Deviation and Variance.vi"("X"=w435) -> ("variance"=w438:dbl)  [unwired: 1 in, 2 out]
        n152 = Divide(x=w437, y=w439) -> (x/y=→"Stiffness_B1X":dbl)
        n153 = Divide(x=w437, y=w438) -> (x/y=→"Stiffness_B1Y":dbl)
      }
    }
    n154 = case shown="True" "Reset" {
      frame False {
      }
      frame True {
        w420 = 0.0 ("QPD_x")
        n155 = local write "QPD_x"(w420) -> ()
        n156 = local write "QPD_y"(w420) -> ()
      }
    }
    n157 = case shown="False" "ON" {
      tunnel: w324 -> [w424 w431]
      tunnel: w323 -> [w426 w434]
      tunnel: [w425 w432] -> w321
      tunnel: [w423 w429] -> w310
      tunnel: w308 -> [w421 w428]
      tunnel: [w421 w428] -> w307
      frame False {
        n158 = local read "QPD_x"() -> (w427:dbl)
        n159 = local read "QPD_y"() -> (w422:dbl)
        n160 = Subtract(x=w426, y=w427) -> (x-y=w425:waveform(dbl))
        n161 = Subtract(x=w424, y=w422) -> (x-y=w423:waveform(dbl))
      }
      frame True {
        n162 = call <vilib>:"Std Deviation and Variance.vi"("X"=w434) -> ("mean"=w433:dbl)  [unwired: 1 in, 2 out]
        "QPD_x" <- w433
        n163 = call <vilib>:"Std Deviation and Variance.vi"("X"=w431) -> ("mean"=w430:dbl)  [unwired: 1 in, 2 out]
        "QPD_y" <- w430
        n164 = Subtract(x=w434, y=w433) -> (x-y=w432:waveform(dbl))
        n165 = Subtract(x=w431, y=w430) -> (x-y=w429:waveform(dbl))
      }
    }
    "B1X" <- w321
    "B1Y" <- w310
    "B1S" <- w307
    n166 = case shown="True" "Clear" {
      frame False {
        # "Do not manipulate the chart histories if the user has not pressed Clear."
      }
      frame True {
        w419 = waveform(dbl)[] [] ("History Data")
        # "Clear the chart histories when the user clicks Clear."
        n167 = property on="B1X" class="WFChart (strict)"("History Data"=w419) -> ()  [unwired: 2 in, 2 out]
        n168 = property on="B1Y" class="WFChart (strict)"("History Data"=w419) -> ()  [unwired: 2 in, 2 out]
        n169 = property on="B1S" class="WFChart (strict)"("History Data"=w419) -> ()  [unwired: 2 in, 2 out]
        n170 = property on="PZTX" class="WFChart (strict)"("History Data"=w419) -> ()  [unwired: 2 in, 2 out]
        n171 = property on="PZTY" class="WFChart (strict)"("History Data"=w419) -> ()  [unwired: 2 in, 2 out]
        n172 = property on="PZTZ" class="WFChart (strict)"("History Data"=w419) -> ()  [unwired: 2 in, 2 out]
        n173 = property on="T1X" class="WFChart (strict)"("History Data"=w419) -> ()  [unwired: 2 in, 2 out]
        n174 = property on="T1Y" class="WFChart (strict)"("History Data"=w419) -> ()  [unwired: 2 in, 2 out]
        n175 = property on="T1Y 2" class="WFChart (strict)"("History Data"=w419) -> ()  [unwired: 2 in, 2 out]
      }
    }
    n176 = Unbundle By Name(w321) -> ("Y"=w320:dbl[])
    n177 = Unbundle By Name(w310) -> ("Y"=w319:dbl[])
    n178 = call <vilib>:"Std Deviation and Variance.vi"("X"=w320) -> ("mean"=w334:dbl)  [unwired: 1 in, 2 out]
    n179 = call <vilib>:"Std Deviation and Variance.vi"("X"=w319) -> ("mean"=w333:dbl)  [unwired: 1 in, 2 out]
    n180 = case shown="True" "BXY" {
      tunnel: w320 -> [_ w470]
      tunnel: w319 -> [_ w471]
      frame False {
      }
      frame True {
        n181 = Bundle("Y"=w470, "Y"=w471) -> (→"B1XY":cluster{"Y":dbl[], "Y":dbl[]})  [unwired: 1 in]
      }
    }
    n182 = Multiply(x=w333, y="B1Y_stiffness") -> (x*y=w330:dbl)
    "Fy" <- w330
    n183 = Multiply(x=w334, y="B1X_stiffness") -> (x*y=w331:dbl)
    "Fx" <- w331
    n184 = global write "Feedback.vi" "Fy"(w330) -> ()
    n185 = global write "Feedback.vi" "Fx"(w331) -> ()
  }
  n186 = while {
    tunnel: w3 -> [w478]
    tunnel: [w474] -> w22
    shift-right: [w477] -> w13
    shift-left: w20 -> [w479]
    stop <- w473 stop-if-true
    # "Event Handling Loop"
    n187 = Wait (ms)(milliseconds to wait=u32 100) -> ()  [unwired: 1 out]
    n188 = event shown="[2] \"Stop_Acquire\": Value Change" {
      selector: w479 -> [_ _ _ _ _ _ _ _ _]
      dyn-events: [_ _ _ _ _ _ _ _ _] -> w477
      timeout: _ -> [_ _ _ _ _ _ _ _ _]
      tunnel: [_ _ _ _ _ _ _ _ TRUE ("Discard?")] -> w473
      tunnel: w478 -> [w481 w485 w490 w494 w497 w500 w504 w510 w511]
      tunnel: [w483 w487 w489 _ w496 w503 _ w505 _] -> w475
      tunnel: [w480 w484 w488 w493 w495 w499 w504 w506 w511] -> w476
      event "Settings": Value Change {
        n189 = event-data() -> ()  [unwired: 1 in, 1 out]
        n190 = call-poly "Enqueue Message.vi"("Message"="Launch Settings Dialog", "Message Queue"=w481) -> ("error out"=w483:errorcluster, "dup Message Queue"=w480:refnum<queue>)  [unwired: 8 in]
      }
      event "Acquire": Value Change {
        n191 = event-data() -> ()  [unwired: 1 in, 1 out]
        n192 = call-poly "Enqueue Message.vi"("Message"="Acquire", "Message Queue"=w485) -> ("error out"=w487:errorcluster, "dup Message Queue"=w484:refnum<queue>)  [unwired: 8 in]
      }
      event "Stop_Acquire": Value Change {
        n193 = event-data() -> ()  [unwired: 1 in, 1 out]
        n194 = call-poly "Enqueue Message.vi"("Message"="Stop_Acquire", "Message Queue"=w490) -> ("error out"=w489:errorcluster, "dup Message Queue"=w488:refnum<queue>)  [unwired: 8 in]
      }
      event "Log": Value Change {
        n195 = event-data() -> ()  [unwired: 1 in, 1 out]
        n196 = call-poly "Enqueue Message.vi"("Message"="Log", "Message Queue"=w494) -> ("dup Message Queue"=w493:refnum<queue>)  [unwired: 8 in, 1 out]
      }
      event "Stop_Log": Value Change {
        (unwired) FALSE
        n197 = event-data() -> ()  [unwired: 1 in, 1 out]
        n198 = call-poly "Enqueue Message.vi"("Message"="Stop_Log", "Message Queue"=w497) -> ("error out"=w496:errorcluster, "dup Message Queue"=w495:refnum<queue>)  [unwired: 8 in]
      }
      event "Exit": Value Change; Panel Close {
        w501 = TRUE  # Priority Message
        # "The UI Message Loop handles sending the Exit message to other loops."
        n199 = event-data() -> ()  [unwired: 1 in, 1 out]
        n200 = call-poly "Enqueue Message.vi"("Priority Message? (F)"=w501, "Message"="Exit", "Message Queue"=w500) -> ("error out"=w503:errorcluster, "dup Message Queue"=w499:refnum<queue>)  [unwired: 7 in]
      }
      event Application Instance Close {
        n201 = event-data() -> ()  [unwired: 1 in, 1 out]
      }
      event Panel Close? {
        # "Send the 'Confirm Quit' message if the user closes the panel of the VI. Discard the event so the 'Confirm Quit' message has a chance to run."
        n202 = event-data() -> ()  [unwired: 1 in, 1 out]
        n203 = call-poly "Enqueue Message.vi"("Priority Message? (F)"=TRUE, "Message"="Confirm Quit", "Message Queue"=w510) -> ("error out"=w505:errorcluster, "dup Message Queue"=w506:refnum<queue>)  [unwired: 7 in]
        n204 = event-data("Discard?"=TRUE) -> ()  [unwired: 1 in, 1 out]
      }
      event User Event {
        # "The Message Handling Loop processed an \"Exit\" message, which fired this event to stop the Event Handling Loop."
        n205 = event-data() -> ()  [unwired: 1 in, 1 out]
        n206 = local write item#4("Exit" ("Exit String")) -> ()
      }
    }
    n207 = call "Error Handler - Event Handling Loop.vi"("error in (no error)"=w475, "Message Queue"=w476) -> ("dup error in"=w474:errorcluster)  [unwired: 8 in, 1 out]
  }
  n208 = call "Acquisition Message Loop.vi"("error in (no error)"=w4, "Data Queue"=w2, "Data Notifier"=w1, "Message Queues"=w16) -> ("error out"=w18:errorcluster)  [unwired: 7 in]
  n209 = call "Logging Message Loop.vi"("error in (no error)"=w4, "Data Queue"=w2, "Message Queues"=w16) -> ("error out"=w15:errorcluster)  [unwired: 8 in]
  n210 = Unregister For Events(event registration refnum=w13, error in=w22) -> (error out=w14:errorcluster)
  n211 = Merge Errors(w14, w23, w18, w15) -> (w21:errorcluster)
  n212 = call "Destroy User Event - Stop.vi"("error in (no error)"=w21, "User Event - Stop"=w19) -> ("error out"=w7:errorcluster)  [unwired: 9 in]
  n213 = disable-structure shown="RUN_TIME_ENGINE==True" {
    disable-tunnel: w7 -> [_ _]
    frame condition #0 {
      # "Call Quit LabVIEW if running as a built application."
      n214 = Quit LabVIEW() -> ()  [unwired: 1 in]
    }
    frame condition #1 (active) {
    }
  }
